vi "Controller Event.vi"() -> ()   [LabVIEW 2021]
uses:
  <vilib>/MakerHub/PS4-Controller/Private/Type Defs/Indicators/Controller.ctl
  <vilib>/MakerHub/PS4-Controller/Private/Type Defs/Indicators/Square.ctl
  <vilib>/MakerHub/PS4-Controller/Private/Type Defs/Indicators/X.ctl
  <vilib>/MakerHub/PS4-Controller/Private/Type Defs/Indicators/Circle.ctl
  <vilib>/MakerHub/PS4-Controller/Private/Type Defs/Indicators/Triangle.ctl
  <vilib>/MakerHub/PS4-Controller/Private/Type Defs/Indicators/L1.ctl
  <vilib>/MakerHub/PS4-Controller/Private/Type Defs/Indicators/R1.ctl
  <vilib>/MakerHub/PS4-Controller/Private/Type Defs/Indicators/Share.ctl
  <vilib>/MakerHub/PS4-Controller/Private/Type Defs/Indicators/Options.ctl
  <vilib>/MakerHub/PS4-Controller/Private/Type Defs/Indicators/PS.ctl
  <vilib>/MakerHub/PS4-Controller/Private/Type Defs/Indicators/Pad_Button.ctl
  <vilib>/MakerHub/PS4-Controller/Private/Type Defs/Indicators/Dpad.ctl
  <vilib>/MakerHub/PS4-Controller/Private/Type Defs/Indicators/Slider.ctl
  <vilib>/MakerHub/PS4-Controller/Public/Open First Controller.vi
  <vilib>/MakerHub/PS4-Controller/LMH-PS4.lvlib
panel:
  out "Checkbox":bool
  out "error out":errorcluster
  in  "Stop Button":bool
  out "PS4 Controller":T1={"Square Button"=FALSE, "X Button"=FALSE, "Circle Button"=FALSE, "Triangle Button"=FALSE, "L1"=FALSE, "R1"=FALSE, "Share Button"=FALSE, "Options Button"=FALSE, "PS Button"=FALSE, "Pad Button"=FALSE, "D-Pad"=5, "L2"=0, "R2"=0, "Thumbstick_Left"={[], []}, "Thumbstick_Right"={[], []}} {"R2" scale=-32768.0..32767.0; "L2" scale=-32768.0..32767.0}
  out "String":string
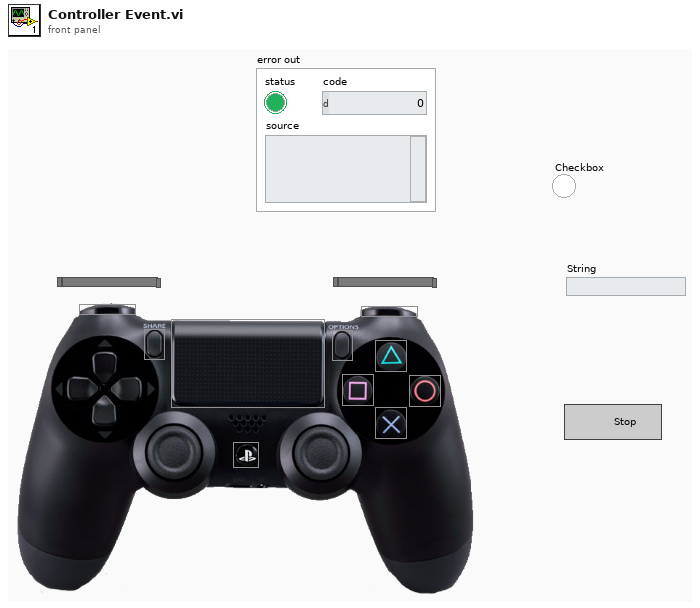
[diagram p1: front panel]
types:
  T1 = typedef "LMH-PS4.lvlib/Controller.ctl" = cluster{"Square Button":T2, "X Button":T3, "Circle Button":T4, "Triangle Button":T5, "L1":T6, "R1":T7, "Share Button":T8, "Options Button":T9, "PS Button":T10, "Pad Button":T11, "D-Pad":T12, "L2":T13, "R2":T13, "Thumbstick_Left":cluster{i32[], i32[]}, "Thumbstick_Right":cluster{i32[], i32[]}}
  T2 = typedef "LMH-PS4.lvlib/Square.ctl" = bool
  T3 = typedef "LMH-PS4.lvlib/X.ctl" = bool
  T4 = typedef "LMH-PS4.lvlib/Circle.ctl" = bool
  T5 = typedef "LMH-PS4.lvlib/Triangle.ctl" = bool
  T6 = typedef "LMH-PS4.lvlib/L1.ctl" = bool
  T7 = typedef "LMH-PS4.lvlib/R1.ctl" = bool
  T8 = typedef "LMH-PS4.lvlib/Share.ctl" = bool
  T9 = typedef "LMH-PS4.lvlib/Options.ctl" = bool
  T10 = typedef "LMH-PS4.lvlib/PS.ctl" = bool
  T11 = typedef "LMH-PS4.lvlib/Pad_Button.ctl" = bool
  T12 = typedef "LMH-PS4.lvlib/Dpad.ctl" = u16
  T13 = typedef "LMH-PS4.lvlib/Slider.ctl" = i32
  T14 = typedef "LMH-PS4.lvlib/PS4 Controller Ref.ctl" = cluster{"Controller Ref":refnum<k1>, "Worker Ref":refnum<vi>, "PS4 Events Ref":refnum<event-registration>}
  T15 = typedef "LMH-PS4.lvlib/Axis.ctl" = cluster{"Left Thumbstick":cluster{"X Axis":i32, "Y Axis":i32}, "Right Thumbstick":cluster{"X Axis":i32, "Y Axis":i32}, "L2":i32, "R2":i32, "D-Pad":T16}
  T16 = typedef "LMH-PS4.lvlib/DPad Enum.ctl" = enum16{"Idle", "Up", "Up / Right", "Right", "Down / Right", "Down", "Down / Left", "Left", "Up / Left"}
  T17 = typedef "LMH-PS4.lvlib/Buttons.ctl" = cluster{"Square":bool, "X":bool, "Circle":bool, "Triangle":bool, "L1":bool, "R1":bool, "L2":bool, "R2":bool, "Share":bool, "Options":bool, "Left Thumbstick":bool, "Right Thumbstick":bool, "Playstation Button":bool, "Pad":bool}
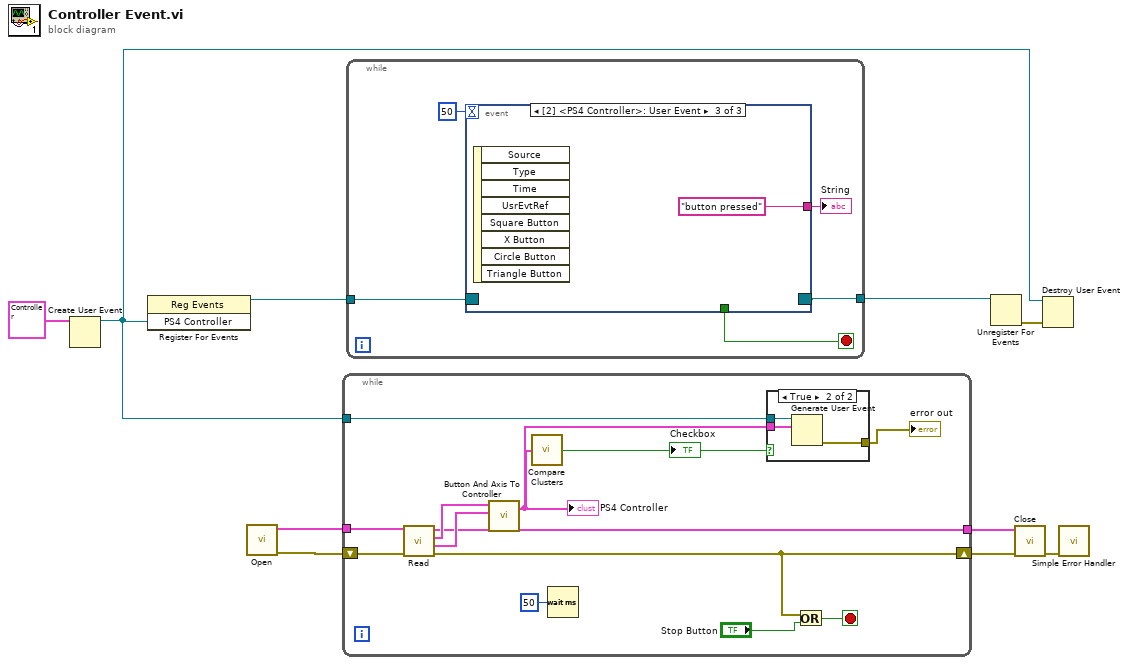
[diagram p0: block diagram]
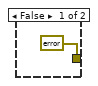
[diagram p2: hidden frame]
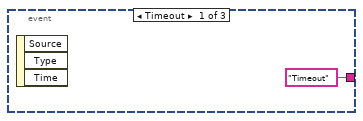
[diagram p3: hidden frame]
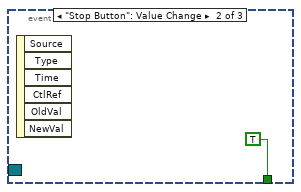
[diagram p4: hidden frame]
diagram:
  n1 = Create User Event(user event datatype=T1 {"Square Button"=FALSE, "X Button"=FALSE, "Circle Button"=FALSE, "Triangle Button"=FALSE, "L1"=FALSE, "R1"=FALSE, "Share Button"=FALSE, "Options Button"=FALSE, "PS Button"=FALSE, "Pad Button"=FALSE, "D-Pad"=5, "L2"=0, "R2"=0, "Thumbstick_Left"={[], []}, "Thumbstick_Right"={[], []}} ("PS4 Controller")) -> (user event=w1:refnum<user-event>)  [unwired: 1 in, 1 out]
  n2 = register-events(w1) -> (reference out=w10:refnum<event-registration>)  [unwired: 2 in, 1 out]
  n3 = call-poly <vilib>:"Open.vi"() -> ("Error Out"=w4:errorcluster, "PS4 Controller Ref"=w3:T14)  [unwired: 9 in, 1 out]
  n4 = while {
    shift-right: [w20] -> w7
    shift-left: w4 -> [w17]
    tunnel: [w19] -> w5
    tunnel: w3 -> [w18]
    tunnel: w1 -> [w15]
    stop <- w21 stop-if-true
    n5 = call <vilib>:"Read.vi"("Error In"=w17, "PS4 Controller Ref"=w18) -> ("Error Out"=w20:errorcluster, "All Axis"=w23:T15, "Buttons"=w22:T17, "PS4 Controller Ref"=w19:T14)  [unwired: 6 in]
    n6 = call <vilib>:"Button And Axis To Controller.vi"("All Axis"=w23, "Buttons"=w22) -> ("PS4 Controller"=w12:T1)  [unwired: 5 in]
    "PS4 Controller" <- w12
    n7 = call "Compare Clusters.vi"("PS4 Controller"=w12) -> ("Checkbox"=w11:bool)
    "Checkbox" <- w11
    n8 = Wait (ms)(milliseconds to wait=u32 50) -> ()  [unwired: 1 out]
    n9 = case shown="True" w11 {
      tunnel: w15 -> [_ w27]
      tunnel: w12 -> [_ w26]
      tunnel: [errorcluster {"status"=FALSE, "code"=0, "source"=""} ("error out") w25] -> w14
      frame False {
      }
      frame True {
        n10 = Generate User Event(user event=w27, event data cluster=w26) -> (error out=w25:errorcluster)  [unwired: 2 in, 1 out]
      }
    }
    "error out" <- w14
    n11 = Or(x=w20, y="Stop Button") -> (x .or. y?=w21:bool)
  }
  n12 = while {
    tunnel: w10 -> [w32]
    tunnel: [w29] -> w8
    stop <- w28 stop-if-true
    n13 = event shown="[2] <PS4 Controller>: User Event" {
      selector: w32 -> [_ _ _]
      dyn-events: [_ _ _] -> w29
      timeout: 50 -> [_ _ _]
      tunnel: ["Timeout" ("String") _ "button pressed" ("String")] -> w31
      tunnel: [_ TRUE ("Stop Button") _] -> w28
      event Timeout {
        n14 = event-data() -> ()  [unwired: 1 in, 3 out]
      }
      event "Stop Button": Value Change {
        n15 = event-data() -> ()  [unwired: 1 in, 6 out]
      }
      event User Event {
        n16 = event-data() -> ()  [unwired: 1 in, 8 out]
      }
    }
    "String" <- w31
  }
  n17 = Unregister For Events(event registration refnum=w8) -> (error out=w9:errorcluster)  [unwired: 1 in]
  n18 = call <vilib>:"Close.vi"("Error In"=w7, "PS4 Controller Ref"=w5) -> ("Error Out"=w6:errorcluster)  [unwired: 9 in]
  n19 = Destroy User Event(user event=w1, error in=w9) -> ()  [unwired: 1 out]
  n20 = call <vilib>:"Simple Error Handler.vi"("error in (no error)"=w6) -> ()  [unwired: 4 in, 5 out]
